vi "Anti-Tip.vi"() -> ()   [LabVIEW 2014]
uses:
  Begin/Global RefNums.vi
  Begin/Global Variables.vi
  _Dependencies/NavX/navX-MXP IMU.lvlib
panel:
  in  "Min Roll":dbl=-12.0
  in  "Min Pitch":dbl=-9.0
  in  "Max Roll":dbl=7.0
  in  "Max Pitch":dbl=6.0
  in  "Buffer":dbl=5.0
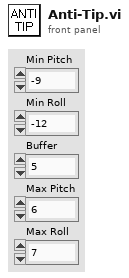
[diagram p1: front panel]
types:
  T1 = typedef "navX-MXP IMU.lvlib/navX Device TypeDef.ctl" = cluster{"navX Interface Protocol":T2, "navX Interface Protocol TypeDefs":cluster{"SPIDevRef":T3, "I2CDevRef":T6}, "navX System Information":cluster{"Board Information":T8, "Status":T9, "Offsets":T13}, "navX Common Information":cluster{"Update Rate (4Hz-60Hz)":T14, "refnum name":string, "error":errorcluster}}
  T2 = typedef "navX-MXP IMU.lvlib/navX Interface Protocol.ctl" = enum16{"SPI", "I2C"}
  T3 = typedef "WPI_SPIDevRef.ctl" = cluster{"DevStatus":errorcluster, "Handle":i32, "Controller":T4, "SPI Bus":T5}
  T4 = typedef "FPGA_TypedefDigitalModule.ctl" = enum16{"Controller 1"}
  T5 = typedef "spi_bus.ctl" = enum16{"SPI On-Board, CS0", "SPI On-Board, CS1", "SPI On-Board, CS2", "SPI On-Board, CS3", "SPI MXP", "Invalid"}
  T6 = typedef "WPI_I2CDevRef.ctl" = cluster{"DevStatus":errorcluster, "Controller":T4, "Device Address":u8, "Handle":i32, "I2C Bus":T7}
  T7 = typedef "i2c_bus.ctl" = enum16{"I2C On-Board", "I2C MXP", "Invalid"}
  T8 = typedef "navX-MXP IMU.lvlib/navX Board Information.ctl" = cluster{"WhoAmI (50 | 0x32)":u8, "Board Revision":u8, "Firmware Major Version":u8, "Firmware Minor Version":u8}
  T9 = typedef "navX-MXP IMU.lvlib/navX Status Data.ctl" = cluster{"Update Rate Hz":u8, "Accelerometer Full-Scale Range":u8, "Gyro Full-Scale Range":u16, "NAVX_OP_STATUS":T10, "NAVX_CAL_STATUS":T11, "NAVX_SELFTEST_STATUS":u8, "NAVX_SENSOR_STATUS":T12}
  T10 = typedef "navX-MXP IMU.lvlib/navX NAVX_OP_STATUS.ctl" = u8
  T11 = typedef "navX-MXP IMU.lvlib/navX NAVX_CAL_STATUS.ctl" = u8
  T12 = typedef "navX-MXP IMU.lvlib/navX NAVX_SENSOR_STATUS.ctl" = cluster{"MOVING":bool, "YAW_STABLE":bool, "MAG_DISTURBANCE":bool, "ALTITUDE_VALID":bool, "SEALEVEL_PRESS_SET":bool, "FUSED_HEADING_VALID":bool}
  T13 = typedef "navX-MXP IMU.lvlib/navX Offsets Data.ctl" = cluster{"Yaw":dbl, "Quat W":dbl, "Quat X":dbl, "Quat Y":dbl, "Quat Z":dbl}
  T14 = typedef "navX-MXP IMU.lvlib/navX Update Rate.ctl" = u8
  T15 = typedef "navX-MXP IMU.lvlib/navX YPRH Data.ctl" = cluster{"Yaw":dbl, "Pitch":dbl, "Roll":dbl, "Heading":dbl}
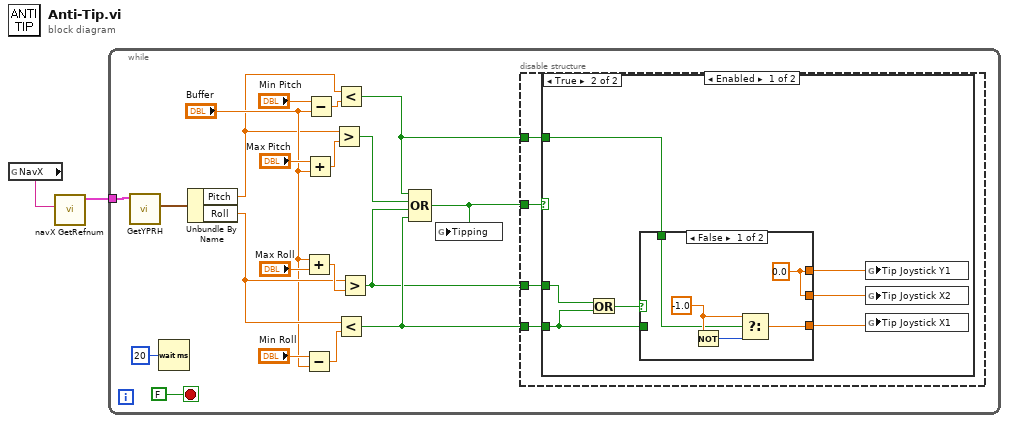
[diagram p0: block diagram]
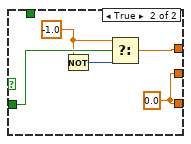
[diagram p3: hidden frame]
diagram:
  n1 = global read "Global RefNums.vi" "NavX"() -> (w2:string)
  n2 = call "navX GetRefnum.vi"("refnum name"=w2) -> ("navX Device TypeDef"=w1:T1)  [unwired: 9 in, 1 out]
  n3 = while {
    tunnel: w1 -> [w7]
    stop <- FALSE stop-if-true
    n4 = call "GetYPRH.vi"("navX Device TypeDef"=w7) -> ("YPRH"=w6:T15)  [unwired: 8 in, 2 out]
    n5 = Wait (ms)(milliseconds to wait=u32 20) -> ()  [unwired: 1 out]
    n6 = Unbundle By Name(w6) -> ("Pitch"=w10:dbl, "Roll"=w17:dbl)
    n7 = Add(x="Buffer", y="Max Roll") -> (x+y=w18:dbl)
    n8 = Subtract(x="Min Roll", y="Buffer") -> (x-y=w16:dbl)
    n9 = Add(x="Max Pitch", y="Buffer") -> (x+y=w19:dbl)
    n10 = Subtract(x="Min Pitch", y="Buffer") -> (x-y=w12:dbl)
    n11 = Greater?(x=w10, y=w19) -> (0:w11:bool)
    n12 = Less?(x=w10, y=w12) -> (x < y?=w5:bool)
    n13 = Less?(x=w17, y=w16) -> (x < y?=w9:bool)
    n14 = Greater?(x=w17, y=w18) -> (0:w8:bool)
    n15 = Compound Arithmetic op=OR(w5, w11, w8, w9) -> (w4:bool)
    n16 = global write "Global Variables.vi" "Tipping"(w4) -> ()
    n17 = disable-structure shown="Enabled" {
      disable-tunnel: w4 -> [w26 _]
      disable-tunnel: w9 -> [w25 _]
      disable-tunnel: w8 -> [w24 _]
      disable-tunnel: w5 -> [w23 _]
      frame Enabled {
        n18 = case shown="True" w26 {
          tunnel: w25 -> [_ w31]
          tunnel: w24 -> [_ w33]
          tunnel: w23 -> [_ w27]
          frame False {
          }
          frame True {
            n19 = Or(x=w33, y=w31) -> (x .or. y?=w32:bool)
            n20 = case shown="False" w32 {
              tunnel: w31 -> [_ w43]
              tunnel: [w34 w40] -> w30
              tunnel: [w35 w40] -> w29
              tunnel: [w35 w39] -> w28
              tunnel: w27 -> [w36 _]
              frame False {
                w38 = -1.0 ("t")
                w35 = 0.0 ("t")
                n21 = Not(x=w38) -> (.not. x?=w37:u32)
                n22 = Select(t=w38, s=w36, f=w37) -> (s? t:f=w34:dbl)
              }
              frame True {
                w40 = 0.0 ("t")
                w42 = -1.0 ("t")
                n23 = Not(x=w42) -> (.not. x?=w41:u32)
                n24 = Select(t=w42, s=w43, f=w41) -> (s? t:f=w39:dbl)
              }
            }
            n25 = global write "Global Variables.vi" "Tip Joystick Y1"(w28) -> ()
            n26 = global write "Global Variables.vi" "Tip Joystick X2"(w29) -> ()
            n27 = global write "Global Variables.vi" "Tip Joystick X1"(w30) -> ()
          }
        }
      }
      frame Disabled {
      }
    }
  }
